vi "Write File.vi"(8 "error in":errorcluster, 10 "Data In":refnum<class "Data.lvclass">, 11 "File Obs in":refnum<class "Tim File Observer.lvclass">) -> (0 "error out":errorcluster, 3 "File Obs out":refnum<class "Tim File Observer.lvclass">)   [LabVIEW 2015, in "Tim File Observer.lvclass"]
doc: "Write data to the file specified in File Ref. The default behavior of this VI is to simply write the Data class to a binary file. This VI may be overriden to provide custom functionality."
uses:
  Tim File Observer.lvclass
  Reusable/CRDS/Data/Cell/CRDS Cell Data.lvclass
  CRD/Data/tCRD Data.lvclass
  Devices/Airmar/Data/Airmar Data.lvclass
  Devices/Alicat/Session Based/Data/MC/MC Data.lvclass
  Reusable/Data/Data.lvclass
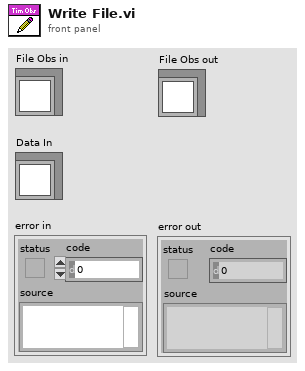
[diagram p1: front panel]
types:
  T1 = cluster{"UTC":timestamp, "Latitude":dbl, "N/S":enum8{"North", "South"}, "Longitude":dbl, "E/W":enum8{"East", "West"}, "GPS Quality":enum16{"Fix not available or invalid", "GPS SPS Mode, fix valid", "Differential GPS, SPS Mode, fix valid", "GPS PPS Mode, fix valid", "Real Time Kinematic", "Float RTK", "Estimated (dead reckoning) Mode", "Manual Input Mode", "Simulator Mode"}, "Number of Satellites":u8, "MSL Altitude":dbl}
  T2 = cluster{"Barometric Pressure":dbl, "Temperature":dbl, "Relative Humidity":dbl, "Dew Point":dbl, "True Wind Direction":dbl, "Magnetic Wind Direction":dbl, "Wind Speed":dbl}
  T3 = typedef "extparam.ctl" = cluster{"Tau":sgl, "Tau0cor":sgl, "ext":sgl, "extCorr":sgl, "stdevTau":sgl, "eTau":sgl, "taucorr":sgl, "Tau0":sgl, "max":sgl}
  T4 = enum16{"Fix not available or invalid", "GPS SPS Mode, fix valid", "Differential GPS, SPS Mode, fix valid", "GPS PPS Mode, fix valid", "Real Time Kinematic", "Float RTK", "Estimated (dead reckoning) Mode", "Manual Input Mode", "Simulator Mode"}
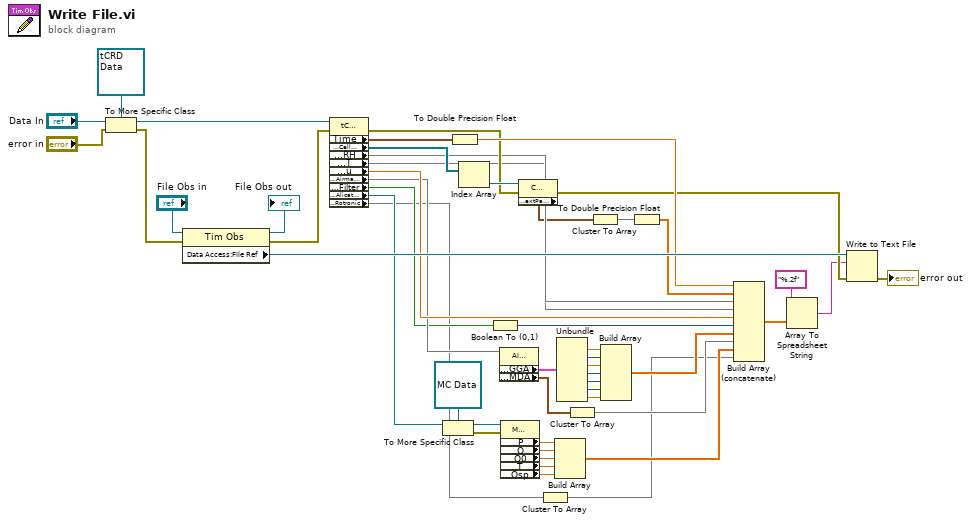
[diagram p0: block diagram]
diagram:
  n1 = To More Specific Class(target class=refnum<class "tCRD Data.lvclass"> refnum ("tCRD Data"), reference="Data In", error in="error in") -> (specific class reference=w47:refnum<class "tCRD Data.lvclass">, error out=w45:errorcluster)
  n2 = property class="Tim Obs"(reference="File Obs in", error in=w45) -> (reference out=→"File Obs out":refnum<class "Tim File Observer.lvclass">, error out=w38:errorcluster, "Data Access:File Ref"=w48:refnum<file>)
  n3 = property class="tCRD Data"(reference=w47, error in=w38) -> (error out=w35:errorcluster, "Time"=w44:timestamp, "Data Access:Cell Data"=w43:refnum<class "CRDS Cell Data.lvclass">[], "Accessors:RH"=w32, "Accessors:T"=w31, "Accessors:u"=w30:sgl, "Accessors:Airmar Data"=w28, "Data Access:Filter"=w26:bool, "Accessors:Alicat Data"=w14:refnum<class "Alicat Data.lvclass">, "Accessors:Rotronic"=w2)  [unwired: 1 out]
  n4 = To More Specific Class(target class=refnum<class "MC Data.lvclass"> refnum ("MC Data"), reference=w14) -> (specific class reference=w13:refnum<class "MC Data.lvclass">, error out=w12:errorcluster)  [unwired: 1 in]
  n5 = To Double Precision Float(number=w44) -> (double precision float=w41:dbl)
  n6 = Index Array(array=w43) -> (element=w42:refnum<class "CRDS Cell Data.lvclass">)  [unwired: 1 in]
  n7 = Boolean To (0,1)(Boolean=w26) -> (0, 1=w25:i16)
  n8 = property class="Airmar Data"(reference=w28) -> ("Accessors:GGA"=w23:T1, "Accessors:MDA"=w27:T2)  [unwired: 1 in, 2 out]
  n9 = property class="MC Data"(reference=w13, error in=w12) -> ("Accessors:P"=w11:sgl, "Accessors:Q"=w10:sgl, "Accessors:Q0"=w9:sgl, "Accessors:T"=w8:sgl, "Accessors:Qsp"=w5:sgl)  [unwired: 2 out]
  n10 = property class="CRDS Cell"(reference=w42, error in=w35) -> (error out=w34:errorcluster, "Data Access:extParam"=w4:T3)  [unwired: 1 out]
  n11 = Cluster To Array(cluster=w2) -> (array=w1:void[])
  n12 = Build Array(w11, w10, w9, w8, w5) -> (w7:sgl[])
  n13 = Unbundle(w23) -> ("Latitude"=w22:dbl, "N/S"=w21:enum8{"North", "South"}, "Longitude"=w20:dbl, "E/W"=w19:enum8{"East", "West"}, "GPS Quality"=w18:T4, "Number of Satellites"=w17:u8, "MSL Altitude"=w16:dbl)  [unwired: 1 out]
  n14 = Cluster To Array(cluster=w27) -> (array=w24:dbl[])
  n15 = Cluster To Array(cluster=w4) -> (array=w3:sgl[])
  n16 = Build Array(w22, w21, w20, w19, w18, w17, w16) -> (w15:dbl[])
  n17 = To Double Precision Float(number=w3) -> (double precision float=w36:dbl[])
  n18 = Build Array (concatenate)(w41, w36, w32, w31, w30, w25, w15, w24, w7, w1) -> (w40:dbl[])
  n19 = Array To Spreadsheet String(array=w40, 3:"%.2f" ("format string")) -> (spreadsheet string=w29:string)  [unwired: 1 in]
  n20 = Write to Text File(file (use dialog)=w48, text=w29, error in=w34) -> (error out=→"error out":errorcluster)  [unwired: 1 in, 2 out]
